vi "Test Executive.vi"(11 "Module Config":T30={"Name"="Test Executive", "Parent Q"=refnum, "Is Child?"=FALSE, "Index"=0, "Dirs"={"Root"=path "C:/MTE", "Config"=path "C:/MTE/Config", "Logs"=path "C:/MTE/Logs", "Reports"=path "C:/ATE/Reports", "App Data"=path "C:/ProgramData/Test Executive"}, "Simulate"=FALSE, "SimCtrl"=refnum}) -> ()   [LabVIEW 2018]
uses:
  <vilib>/KATE/Module/Module Config.ctl
  <vilib>/KATE/Queues/Q.Element.ctl
  <vilib>/KATE/Module/Module.Working Dirs.ctl
  Controls and Type Defs/TestExec.Station ID.ctl
  <vilib>/KATE/SeqMgr/SeqMgr.Result State Enum.ctl
  SubVIs/Metrics/TestExec.Test Result Metric Status.ctl
  Common/Utils/Results/Result.Results Table Record.ctl
  Common/Utils/Errors/Error.Error List Item.ctl
  Common/Utils/Errors/Error.Warning List Item.ctl
  Common/Utils/Results/Result XML/TestResult.SW Item.ctl
  SubVIs/TestExec.Test Result Metric History.ctl
  SubVIs/Metrics/TestExec.Test Result Metric History Item.ctl
  Controls and Type Defs/TestExec.Test Data Directories.ctl
  Common/Utils/TestExec/TestExec.WorkingDir.ctl
  Controls and Type Defs/TestExec.Options Ctrls.ctl
  <vilib>/KATE/Event Log/Event Notification/Event Log.Log Level.ctl
  Common/Utils/Results/Limits/Result.Test Limit Item.ctl
  Common/Utils/Results/Result.Limit Type.ctl
  SubVIs/Options/TestExec.Result Option Selector.ctl
  Controls and Type Defs/TestExec.Barcode PN SN Format Type.ctl
  Common/Utils/Reports/Report.Result FileDataObject.ctl
  <vilib>/KATE/Files/Sync/File.Sync Item Record.ctl
  Common/Utils/Reports/Report.Report File Config Item.ctl
  Common/Utils/Reports/Report.Report File Type.ctl
  <vilib>/KATE/Module/Module.SW Version Info.ctl
  <vilib>/KATE/Module/Window/Window.Task, Action.ctl
  Common/Utils/TestExec/TestExec.Health State Command.ctl
  SubVIs/Mode Manager/Mode Manager.lvclass
  Controls and Type Defs/TestExec.Sequence Info.ctl
  <vilib>/KATE/SeqMgr/SeqMgr.Result Info.ctl
  Controls and Type Defs/TestExec.Health Management Params.ctl
  <vilib>/KATE/SeqMgr/SeqMgr.lvclass
  <vilib>/KATE/Files/Sync/File.Sync.lvclass
  <vilib>/KATE/TCP-IP/Mgr/TCP-IP Mgr.Config.ctl
  Common/Utils/Counters/Step Counter.State Info.ctl
  Common/Utils/Results/Result.Measurement Item.ctl
  Common/Utils/Results/Result.Measurement and Attribute Item Status.ctl
  Common/Utils/Results/Result XML/TestResult.Header Info.ctl
  Common/Utils/Results/Result XML/TestResult.Facility.ctl
  Common/Utils/Results/Result XML/TestResult.Station Info.ctl
  Common/Utils/Results/Result XML/TestResult.HW Item.ctl
  Common/Utils/Results/Result XML/TestResult.Test Run Info.ctl
  Common/Utils/Results/Result XML/TestResult.Test Info.ctl
  Common/Utils/Results/Result XML/TestResult.UUT Result.ctl
  Common/Utils/Results/Result XML/TestResult.Symptom.ctl
  Common/Utils/Results/Result XML/TestResult.Symptom.State.ctl
  Common/Utils/Results/Result XML/TestResult.UUTInfo.ctl
  Common/Utils/Subscription/Subscription.Request Item.ctl
  Common/Utils/Errors/Error.Error Code List.ctl
  Common/Utils/Counters/SubVIs/Step Counter.Action.ctl
  Common/Utils/Results/Result.Attribute.ctl
  Common/Utils/Results/Result.Attribute_EV1.ctl
  Common/Utils/Results/Result XML/TestResult.FullResultData.ctl
  Common/Utils/Results/Result.Report Format Selector.ctl
  Common/Utils/Results/Result.Numeric.ctl
  Common/Utils/Results/Result.Numeric_EV1.ctl
  Common/Utils/TestExec/TestExec.Operating State.ctl
  <vilib>/KATE/Queues/Q.Msg Return Data Container.ctl
  Common/Utils/TestExec/TestExec.Test Start Message to Sta.ctl
  SubVIs/Metrics/TestExec.Test Metric Action Selector.ctl
  <vilib>/KATE/SeqMgr/SeqMgr.Result Control Ref.ctl
  <vilib>/KATE/SeqMgr/SeqMgr.Progress Controls.ctl
  Common/Utils/TestExec/TestExec.Test Launch Params.ctl
  <vilib>/KATE/Event Log/Event Notification/Event Log.Notification Type.ctl
  <vilib>/Utility/config.llb/Read Key (String).vi
  <vilib>/KATE/Config/Stored Controls/Class.SaveCtrls.lvclass
  <vilib>/KATE/Queues/Queue Utils.lvlib
  <vilib>/KATE/Module/Module Utils.lvlib
  <vilib>/KATE/Event Log/Event Log.lvlib
  <vilib>/KATE/Scheduler/Scheduler.lvlib
  <vilib>/KATE/Files/File Utils.lvlib
  <vilib>/KATE/Menu/Menu Utils.lvlib
  <vilib>/KATE/SeqMgr/SeqMgr.lvlib
  <vilib>/KATE/Config/Config Utils.lvlib
  <vilib>/KATE/Controls/Controls.lvlib
  <vilib>/KATE/Graphics/Graphic Utils.lvlib
  <vilib>/KATE/TCP-IP/TCP-IP.lvlib
  <vilib>/KATE/Event Log/Event Notification/Event Notification.lvclass
  <vilib>/KATE/Time/Time Utils.lvlib
  <vilib>/Utility/config.llb/NI_LVConfig.lvlib
  <vilib>/KATE/Config/App Data/Class.AppData.lvclass
  <vilib>/KATE/Files/Rotate/File.Rotate.lvclass
panel:
  in  "Main Tab":enum32{"Operate", "Maint"}(tab)
  in  "PersistCmt":bool caption="Persist"
  in  "Comment At End":bool caption="Prompt"
  out "Route Check":bool caption="SN Route Check"
  out "Duration(HH:MM:SS)":string
  out "Position":string
  out "Remote":bool
  out "Wiggler":bool
  out "StaCnct":bool caption="Connected"
  out "PLC":bool
  out "Status":string
  out "Result Status":T2 {"Code" format="%08d"}
  in  "Start with SN Entry":bool=TRUE caption="Start Test with SN Entry"
  in  "Go to Test Metric Details":bool
  in  "Kill Auto Launch":bool
  out "Repeat Notificaiton":string
  in  "Comment":string
  in  "SN":string
  in  "Test Result Metrics":T3
  in  "Operator":string
  in  "Mode":u16(ring) items=["Production", "Technician", "Gage R&R", "Engineering"]
  out "Station":T4
  out "End Time":timestamp format="%<%X\n%x>T"
  out "Start Time":timestamp format="%<%X\n%x>T"
  out "Simulate Indication":string="Simulating Instruments"
  in  "Funct Tab":T5(tab)
  out "Seq Rslt":string caption="Seq"
  out "SN Rslt":string caption="SN"
  in  "Test Status Tab":T6(tab)
  out "Abort Cnt":i32
  out "Test State":enum32{"Idle", "Running", "Completed"}(tab)
  out "Progress 2":dbl(slide) caption="Progress" scale=0.0..1.0
  out "Test Running 2":bool
  out "Result Status 2":T2 {"Code" format="%08d"}
  out "Yield%":dbl
  out "Error Cnt":i32
  out "Fail Cnt":i32
  out "Pass Cnt":i32
  in  "Filter":string
  in  "Show Only Failures":bool
  out "Results Table":T7[](array[typedef]) caption="Results"
  in  "Auto Scroll":bool=TRUE
  in  "Open Image File":bool
  in  "OperNo":bool
  out "OperPrompt":string caption="Oper Instructions"
  in  "OperOK":bool
  out "OperPict":picture
  in  "Zoom Img":dbl(slide)=1.0 caption="Zoom" min=0.1 max=10.0 step=0.01 scale=0.0..2.0
  in  "Zoom Right":dbl(slide)=1.0 min=0.1 max=10.0 step=0.01 scale=0.0..2.0
  in  "Zoom Left":dbl(slide)=1.0 min=0.1 max=10.0 step=0.01 scale=0.0..2.0
  out "Rigth Image":picture
  out "Left Image":picture
  in  "OperOK 2":bool
  in  "OperNo 2":bool
  in  "Prompt NO":bool
  in  "Prompt YES":bool
  in  "Prompt2_OK":bool
  in  "OperInput Data":string caption="Input Data"
  out "OperPrompt2":string caption="Instructions"
  in  "Test Reset":bool
  in  "ReportEn":T8=1 caption="Reports" items=["Enabled", "Disabled"]
  in  "Test Status Tab Sel":u16(ring) caption="View" items=["Summary", "Results", "Image1", "Image2", "Prompt"]
  out "Equipment List":string[][](table)
  in  "Health Tab":T9(tab)
  in  "Clear Errors and Warnings":bool
  in  "Clear Errors":bool
  in  "Clear Warnings":bool
  out "Warning List":T10[](array[typedef])
  out "Error List":T11[](array[typedef])
  in  "Open Event Log":bool
  in  "Open SW Version File":bool
  out "LastVerCkTime":timestamp caption="Last Version Check"
  out "SW Check Config":T12
  out "RelSWVers":string[][](array[string]) caption="Released SW Versions"
  out "Station SW Versions":T13(array[cluster])
  in  "Enable File Sync":bool=TRUE
  out "FileSyncActive":bool
  in  "Sync Now":bool
  out "Sync Items":T14[](array[typedef])
  in  "Test Metrics Tab":enum32{"Test History", "Test Reports", "Pareto"}(tab)
  in  "Test Cycle Cnt Reset":bool
  out "Total Test Cycles":i32
  in  "Test Metrics Reset":bool
  out "Test History":T15 {"Dur(s)" format="%#.1f"}
  in  "Open RprFldr":cluster{"Open":bool}[](array[cluster])
  in  "Configure Reports":bool
  out "Report Config":T17[](array[typedef]) caption="Name/\nType                                                            Sequence                                                                                             Output Folder"
  out "Pareto":i32[][](array[numeric]) caption="Code                        Count"
  in  "Config Tab":T19(tab)
  out "Force Sync Now":bool
  in  "SyncType":bool caption="Sync Type: Difference(F) or All(T)"
  in  "Set TE Sta Cfg":bool
  out "PLC Running":bool
  in  "Sim Wiggler Start":bool
  in  "TE Opts":T20={"DispDetails"=FALSE, "NotResetSN"=FALSE, "NotValOper"=FALSE, "NotValSN"=FALSE, "DisResults"=FALSE, "StaModule"=FALSE, "EditEQ"=FALSE, "ClrWarn"=FALSE, "ClrErr"=FALSE, "ViewCfg"=FALSE, "SetOpts"=FALSE, "ContOnErr"=FALSE, "ContOnFail"=TRUE, "DisMetrics"=FALSE, "SelSeq"=FALSE, "GenRpt"=FALSE, "DisStartWithSN"=FALSE, "Auto Repeat Seq En"=FALSE, "DataDirEn"=FALSE, "SNRouteCk"=FALSE} caption="TE Options"
  in  "Default Timeout (s)":dbl=1.0
  in  "Show Station Module":bool
  in  "Log Level":T21
  in  "PLC Enable":bool=TRUE
  out "Duration(s)":dbl format="%.2f"
  out "Step":string[](array[string])
  in  "Inc Step":bool
  in  "Pause":bool
  in  "Step Run":bool
  out "Script":string[][](array[string])
  out "StepCnt":i32
  in  "Run Utility":bool
  in  "Utility INI Config File":u16(ring)
  in  "Args":string[](array[string])
  in  "Exe Path":path
  in  "Run Exe":bool
  out "Seq Setup":cluster{"Name":string, "Value":string}[](array[cluster]) caption="Setup:   Name                                Value"
  out "SeqName":string caption="Name"
  out "SeqPN":string caption="PN"
  out "SeqVer":string caption="Version"
  out "Data Dir Config":T22
  out "PN":string
  out "UUT Properties":string[][](array[string])
  out "Variables":string[][](array[string])
  in  "Barcode PN SN Format":T24={"Type"=enum."SN_Only", "Len"=12, "Delimiter"="TAB"}
  out "Image Path":path
  out "Var Subscribe":bool
  in  "LoadLimFile":bool
  out "Limit File Ver":string
  out "Limits":T25[](array[typedef])
  out "Limit File Name":string
  in  "Open Root Folder":bool
  out "Cfg.Dirs":T27
  out "CfgFilePaths":T28
  out "File Data Objs":T29[](array[typedef])
  out "Title":string="Test Executive"
  out "Rev":string="v1.0.0"
  in  "Go to Health Details":bool
  out "Warnings":i32 caption="Counts"
  out "Errors":i32
  out "Health OK":bool
  out "Test Ctrl Tab":enum32{"Idle", "Running", "Completed"}(tab)
  in  "Start":bool
  out "UUT SN Status":string="Enter Operator and SN then click Start."
  in  "Sequence":u16(ring) items=["Test_01", "Test_02", "Test_03", "Test_04", "Test_05", "Test_06", "Test_07", "Test_08", "Test_09"]
  out "Test Running":bool
  out "Progress":dbl(slide) scale=0.0..1.0
  in  "Abort":bool
  out "Failing Status":string="Failing"
  in  "RepeatInt(s)":dbl=3.0 caption="(s)"
  in  "Repeat Seq":bool
  in  "Exit Sta module":bool
  out "StaModule":string
  in  "Leave Maint":bool
  out "Abort Flag":bool
  in  "Create RTF Report":bool
  out "OperCntDwn":dbl caption="Seconds Remaining" format="%#.0f"
  in  "TO_En":bool caption="Enabled"
  out "SW Items":T31[](array[typedef]) caption="This Station SW Items"
  # "Health\nStatus"
  # "Yield = 100% X Pass / (Pass + Fail + Error)"
  # "Ready\nfor Next Test"
  # "Step                                        Name                                                   Value                          Units    LimType       LL            UL           Result        Code                     Description"
  # "Image Prompt"
  # "Name                                                                            PN                                  Version                                   Checked    Wrong Version"
  # "Name                                                                     Version"
  # "Name/Interval(Hours)                                                                       Source/Destination                                                                                       Last Sync                                 Status"
  # "Dur(s)                    Time                               Mode                           Test                                   SN                               Result            Code                                          Description"
  # "Test Report Configuration"
  # "If a sequence name is listed, then the report will be sent to the corresponding folder.\nIf the sequenceis not in the list then the report will be sent to the first folder (the default folder)."
  # "Difference:    Only overwrite difference.\nAll:                    Always over write all."
  # "Sequence Info"
  # "Name                                                       Value"
  # "Name                                                       Value"
  # "String or Special Chars: \n  TAB CR LF EOL(CRLF)"
  # "Name                        Type               LL             UL                Units         FailCode                                     Fail Desc"
  # "Image1 Time Out"
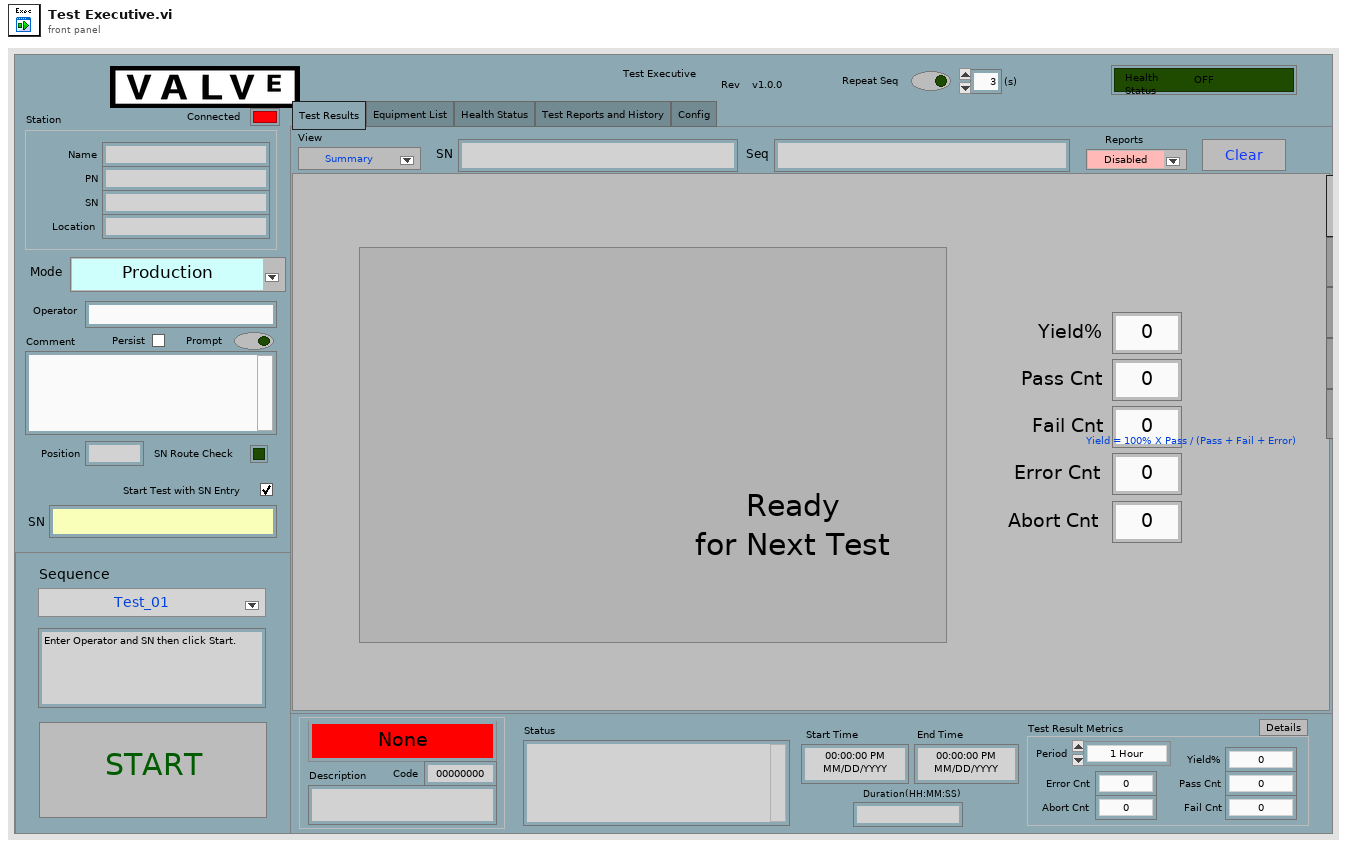
[diagram p1: front panel]
types:
  T1 = typedef "KATE_Lib.lvlib/SeqMgr.lvlib/SeqMgr.Result State Enum.ctl" = enum16{"None", "Passing", "Failing", "PASS", "FAIL", "ABORT", "ERROR"}
  T2 = cluster{"State":T1, "Code":i32, "Description":string}
  T3 = typedef "TestExec.Test Result Metric Status.ctl" = cluster{"Period":enum16{"1 Hour", "4 Hours", "1 Day", "1 Week"}, "Pass Cnt":i32, "Fail Cnt":i32, "Yield%":dbl, "Error Cnt":i32, "Abort Cnt":i32}
  T4 = typedef "TestExec.Station ID.ctl" = cluster{"Name":string, "PN":string, "SN":string, "Location":string}
  T5 = enum32{"Test Results", "Station Control", "Equipment List", "Health Status", "Test Reports and History", "Config"}
  T6 = enum32{"Summary", "Results", "Image1", "Image2", "Prompt"}
  T7 = typedef "Result.Results Table Record.ctl" = cluster{"Cnt":i32, "Step":string, "Category":string, "Name":string, "Value":string, "Units":string, "LimType":string, "LL":string, "UL":string, "Status":string, "Status Color":u32, "Code":i32, "Desc":string}
  T8 = typedef "TestExec.Result Option Selector.ctl" = u16
  T9 = enum32{"Errors/Warnings", "SW Versions", "File Sync", "File Rotation"}
  T10 = typedef "Error.Warning List Item.ctl" = cluster{"Code":i32, "Desc":string, "First":timestamp, "Last":timestamp, "Count":i32}
  T11 = typedef "Error.Error List Item.ctl" = cluster{"Code":i32, "Desc":string, "First":timestamp, "Last":timestamp, "Count":i32}
  T12 = cluster{"Check Interval":dbl, "SW Version List File":path, "Enabled":bool}
  T13 = cluster{"Name":string, "PN":string, "Version":string, bool, bool}[]
  T14 = typedef "KATE_Lib.lvlib/File Utils.lvlib/File.Sync.lvclass/File.Sync Item Record.ctl" = cluster{"Name":string, "Interval":dbl, "Source":path, "Dest":path, "LastSync":timestamp, "Status":string, "Error":bool, "Type":enum16{"Merge", "Match"}}
  T15 = typedef "TestExec.Test Result Metric History.ctl" = T16[]
  T16 = typedef "TestExec.Test Result Metric History Item.ctl" = cluster{"TimeStamp":timestamp, "Dur(s)":dbl, "Time":string, "Mode ":string, "Test ":string, "SN":string, "State":T1, "Code":i32, "Description":string}
  T17 = typedef "Report.Report File Config Item.ctl" = cluster{"Name":string, "Type":T18, "Seq_Dir":cluster{"Sequence":string, "Folder":path}[]}
  T18 = typedef "Report.Report File Type.ctl" = enum16{"CSV_WithConfigAndData", "CSV", "CSV_SummaryResult", "JSON", "JSON_WithFiles", "XLINK", "XLINK_ResultOnly", "SFC1", ""}
  T19 = enum32{"Options", "Script Debug", "Run Util", "Run Exe", "Client Info", "Local Data", "Limits", "Dirs", "File Objs"}
  T20 = typedef "TestExec.Options Ctrls.ctl" = cluster{"DispDetails":bool, "NotResetSN":bool, "NotValOper":bool, "NotValSN":bool, "DisResults":bool, "StaModule":bool, "EditEQ":bool, "ClrWarn":bool, "ClrErr":bool, "ViewCfg":bool, "SetOpts":bool, "ContOnErr":bool, "ContOnFail":bool, "DisMetrics":bool, "SelSeq":bool, "GenRpt":bool, "DisStartWithSN":bool, "Auto Repeat Seq En":bool, "DataDirEn":bool, "SNRouteCk":bool}
  T21 = typedef "KATE_Lib.lvlib/Event Log.lvlib/Event Log.Log Level.ctl" = enum16{"Normal", "Verbose", "Debug0", "Debug1", "Debug2"}
  T22 = typedef "TestExec.Test Data Directories.ctl" = cluster{"Station Data":T23[], "SeqRsltDirs":T23[]}
  T23 = typedef "TestExec.WorkingDir.ctl" = cluster{"Name":string, "Path":path}
  T24 = typedef "TestExec.Barcode PN SN Format Type.ctl" = cluster{"Type":enum16{"SN_Only", "SN_PN_LenDelim", "PN_SN_LenDelim", "SN_PN_StrDelim", "PN_SN_StrDelim"}, "Len":i32, "Delimiter":string}
  T25 = typedef "Result.Test Limit Item.ctl" = cluster{"Name":string, "LimType":T26, "LL":string, "UL":string, "Units":string, "FailCode":i32, "FailDesc":string}
  T26 = typedef "Result.Limit Type.ctl" = enum16{"None", "EQ", "NE", "GT", "LT", "GE", "LE", "GTLT", "GELE", "GELT", "GTLE", "LTGT", "LEGE", "LEGT", "LTGE", "Contains", "NotContains"}
  T27 = typedef "KATE_Lib.lvlib/Module Utils.lvlib/Module.Working Dirs.ctl" = cluster{"Root":path, "Config":path, "Logs":path, "Reports":path, "App Data":path}
  T28 = cluster{"ModeCfg":path, "DataTemp":path, "SW Limits":path, "SW Sequences":path, "Rel_SW":path, "Current Seq Dir":path, "RouteCfg":path, "WorkingCfg":path, "Devcon":path, "ScriptLibDirs":path[], "Archive":path, "LocalData":path}
  T29 = typedef "Report.Result FileDataObject.ctl" = cluster{"Cnt":i32, "Step":string, "Category":string, "Name":string, "Type":string, "File Name":string, "Time":string, "Path":path}
  T30 = typedef "KATE_Lib.lvlib/Module Utils.lvlib/Module Config.ctl" = cluster{"Name":string, "Parent Q":refnum<queue>, "Is Child?":bool, "Index":i32, "Dirs":T27, "Simulate":bool, "SimCtrl":refnum<vi>}
  T31 = typedef "TestResult.SW Item.ctl" = cluster{"Name":string, "PN":string, "Version":string, "Note":string}
  T32 = typedef "KATE_Lib.lvlib/Module Utils.lvlib/Module.SW Version Info.ctl" = cluster{"AppName":string, "Company":string, "Version":string, "Description":string, "PN":string}
  T33 = typedef "KATE_Lib.lvlib/Module Utils.lvlib/Module Sys Info.ctl" = cluster{"Main Q":refnum<queue>, "Exe":bool, "SW Rev":T32, "Self Ref":refnum<vi>, "Main Tab":refnum<vi>, "Pane":refnum<vi>, "Stop":cluster{"Ref":refnum<event-registration>, "Event":refnum<user-event>}, "Cfg":T30, "Services":cluster{"Name":string, "vi ref":refnum<vi>}[], "Menu Ref":refnum<k9>, "CtrlStates":refnum<class "Class.SaveCtrls.lvclass">, "Docs":cluster{"Tags":string[], "Paths":path[]}, "Log":refnum<class "Event Notification.lvclass">, "Test Controls":refnum<vi>[], "Child Modules":cluster{"Name":string, "vi ref":refnum<vi>}[], "SW Items":string[][], "AppData":refnum<class "Class.AppData.lvclass">, "Subscriptions":refnum<class "Subscription.lvclass">}
  T34 = typedef "KATE_Lib.lvlib/TCP-IP.lvlib/TCP-IP Mgr.Config.ctl" = cluster{"IP":string, "Port":u16, "Listener":bool, "Enable":bool}
  T35 = cluster{"Oper":cluster{"OK":bool, "Desc":string}, "SN":cluster{"OK":bool, "Desc":string}, "NoSN":bool, "DefaultSN":string, "SNErr":bool, "SeqEn":enum8{"Enabled", "Disabled", "Disabled and Grayed Out"}}
  T36 = enum8{"Enabled", "Disabled", "Disabled and Grayed Out"}
  T37 = typedef "TestExec.Health State Command.ctl" = enum16{"Update", "Clear All", "Clear Warnings", "Clear Errors", "Set Warning", "Set Error"}
  T38 = typedef "Result.Measurement Item.ctl" = cluster{"Cnt":i32, "Step":string, "Category":string, "Name":string, "Value":string, "Units":string, "LimType":string, "LL":string, "UL":string, "Status":T39, "Code":i32, "Desc":string, "Time":timestamp}
  T39 = typedef "Result.Measurement and Attribute Item Status.ctl" = i32
  T40 = typedef "Step Counter.Action.ctl" = enum16{"Init", "Section Start", "Data +", "Sub Section Start", "Sub Section End", "Get Step"}
  T41 = typedef "TestResult.HW Item.ctl" = cluster{"Name":string, "MFG":string, "PN":string, "SN":string, "SW/FW":string, "Note":string, "Cal_ID":string, "Cal_Type":string, "Cal_Due_Date":timestamp, "Cal_Status":string}
  T42 = cluster{"Config Folder":path, "Seq Folder":path, "Rel SW File":path, "SW Check Int(s)":dbl, "Vers":variant, "SW Check En":bool}
  T43 = typedef "Result.Attribute.ctl" = cluster{"Cnt":i32, "Step":string, "Category":string, "Name":string, "Value":string, "Status":T39, "Code":i32, "Desc":string, "Time":timestamp}
  T44 = typedef "Result.Attribute_EV1.ctl" = cluster{"Cnt":i32, "Step":string, "Category":string, "Name":string, "Value":string, "Status":T39, "Code":i32, "Desc":string}
  T45 = typedef "Result.Report Format Selector.ctl" = enum16{"XML", "CSV", "Xlink XML", "XML with Files", "JSON", "JSON with Files", "RTF", "SFC1"}
  T46 = typedef "TestResult.FullResultData.ctl" = cluster{"#attributes":cluster{"Version":string}, "Station":T47, "Test Run":T48, "Test Sequence":T49, "UUTs":cluster{"UUT":T50[]}}
  T47 = typedef "TestResult.Station Info.ctl" = cluster{"Name":string, "PN":string, "SN":string, "Rev":string, "PC Name":string, "Location":string, "HW_Config":cluster{"HW_Item":T41[]}, "SW_Config":cluster{"SW_Item":T31[]}}
  T48 = typedef "TestResult.Test Run Info.ctl" = cluster{"Operator":string, "Start Time":timestamp, "Duration(s)":dbl, "Mode":string, "Comment":string, "ProcessStep":string}
  T49 = typedef "TestResult.Test Info.ctl" = cluster{"Name":string, "Config":cluster{"Config_Item":cluster{"Name":string, "Value":string}[]}}
  T50 = typedef "TestResult.UUT Result.ctl" = cluster{"Position":string, "Result":T51, "Measurements":cluster{"Measurement":T38[]}, "UUTInfo":T53}
  T51 = typedef "TestResult.Symptom.ctl" = cluster{"Result":T52, "Code":i32, "Description":string}
  T52 = typedef "TestResult.Symptom.State.ctl" = enum16{"Pass", "Fail", "Error", "Aborted", "Completed", "Logged"}
  T53 = typedef "TestResult.UUTInfo.ctl" = cluster{"Product":string, "Desc":string, "PN":string, "SN":string, "Lot":string, "DateCode":string, "AltID":string, "Revision":string, "Properties":cluster{"Property":cluster{"Name":string, "Value":string}[]}}
  T54 = typedef "TestExec.Operating State.ctl" = cluster{"Test State":enum32{"Idle", "Running", "Completed"}, "Result":T1, "Sequence":string, "Sequences":string[], "SN":string, "Position":string}
  T55 = typedef "KATE_Lib.lvlib/Queue Utils.lvlib/Q.Msg Return Data Container.ctl" = cluster{"SeqNum":i32, "Data":variant, "Error":errorcluster}
  T56 = typedef "TestExec.Test Start Message to Sta.ctl" = cluster{"Test Name":string, "Start Time":timestamp, "UUT SN":string}
  T57 = typedef "KATE_Lib.lvlib/Module Utils.lvlib/Window.Task, Action.ctl" = enum16{"Resize()", "Show Panel(Bool)", "Show Scroll Bars(Bool)", "Dock to SubPanel(SubPanel Ref)", "Undock from SubPanel()", "Return to SubPanel()", "Go To Maint Tab()", "Show Maint Tab(Bool)", "Open Block Diagram()"}
  T58 = typedef "Subscription.Request Item.ctl" = cluster{"Name":string, "Msg":T59}
  T59 = typedef "KATE_Lib.lvlib/Queue Utils.lvlib/Q.Element.ctl" = cluster{"Cmd":string, "Sub":string, "Data1":variant, "Data2":variant}
  T60 = typedef "TestExec.Test Metric Action Selector.ctl" = enum16{"Append", "Get Metrics", "Reset", "Load", "Save"}
  T61 = typedef "TestExec.Test Launch Params.ctl" = cluster{"Sequence":string, "SN":string, "Pos":string}
  T62 = cluster{"Config_Item":cluster{"Name":string, "Value":string}[]}
  T63 = typedef "KATE_Lib.lvlib/SeqMgr.lvlib/SeqMgr.Result Info.ctl" = cluster{"State":T1, "Code":i32, "Description":string}
  T64 = typedef "KATE_Lib.lvlib/Event Log.lvlib/Event Log.Notification Type.ctl" = enum16{"Normal", "Warning", "Error", "Success"}
  T65 = typedef "TestExec.Health Management Params.ctl" = cluster{"Warnings":i32, "Errors":i32, "LastVerCk":dbl, "VerCkInterval":dbl, "SW Check En":bool, "Init":bool, "LastVerListCk":dbl}
  T66 = typedef "TestExec.Sequence Info.ctl" = cluster{"Name":string, "Path":path}
  T67 = cluster{"ModeCfg":path, "DataTemp":path, "SW Limits":path, "SW Sequences":path, "Rel_SW":path, "CurSeqDir":path, "RouteCfg":path, "WorkingCfg":path, "Devcon":path, "ScriptLibDirs":path[], "Archive":path, "LocalData":path}
  T68 = cluster{"Child Modules":cluster{"VI Ref":refnum<vi>, "Name":string}[]}
  T69 = cluster{"Limits":variant, "Limit File":string, "Limit Ver":string, "RsltCodes":variant, "Rslt Code File":string, "Rslt Code Ver":string, "Default Seq":i32, "FaultPrefix":i32, "UUTRoutes":string[], "DisableRouteCk":bool, "StaVer":i32, "SN Valid":bool, "ReqVars":bool, "Product":string, "ProcessStep":string, "FileSyncMaster":path, "CmtPrmpt":bool}
  T70 = typedef "TestResult.Header Info.ctl" = cluster{"#attributes":cluster{"Version":string}, "Facility":T71, "Station":T47, "Test Run":T48, "Test Sequence":T49}
  T71 = typedef "TestResult.Facility.ctl" = cluster{"Name":string, "Location":string}
  T72 = typedef "Step Counter.State Info.ctl" = cluster{"Level":i32, "Cnts":i32[], "Step":string, "Cntr":i32}
  T73 = cluster{"Lnch":bool, "SeqTimer":dbl, "TimeOut(s)":dbl, "ModeMgr":refnum<class "Mode Manager.lvclass">, "CfgFilePaths":cluster{"ModeCfg":path, "DataTemp":path, "SW Limits":path, "SW Sequences":path, "Rel_SW":path, "CurSeqDir":path, "RouteCfg":path, "WorkingCfg":path, "Devcon":path, "ScriptLibDirs":path[], "Archive":path, "LocalData":path}, "Data Dirs":T22, "StaApp":string, "App":cluster{"Child Modules":cluster{"VI Ref":refnum<vi>, "Name":string}[]}, "Sequences":T66[], "PreTestCk":cluster{"Oper":cluster{"OK":bool, "Desc":string}, "SN":cluster{"OK":bool, "Desc":string}, "NoSN":bool, "DefaultSN":string, "SNErr":bool, "SeqEn":enum8{"Enabled", "Disabled", "Disabled and Grayed Out"}}, "Seq":string[][], "SeqMgr":refnum<class "SeqMgr.lvclass">, "Health":T65, "ResultState":T63, "SW_Vers":variant, "Repeat(s)":dbl, "DisableResults":bool, "SectCtr":T72, "Data":cluster{"FileObjs":T29[], "Meas":T38[]}, "ResultError":errorcluster, "RptHdr":T70, "RptUUT":T50, "Lists":cluster{"Limits":variant, "Limit File":string, "Limit Ver":string, "RsltCodes":variant, "Rslt Code File":string, "Rslt Code Ver":string, "Default Seq":i32, "FaultPrefix":i32, "UUTRoutes":string[], "DisableRouteCk":bool, "StaVer":i32, "SN Valid":bool, "ReqVars":bool, "Product":string, "ProcessStep":string, "FileSyncMaster":path, "CmtPrmpt":bool}, "TestCanceled":bool, "Opts":T20, "UUT Dir":path, "Funct":cluster{"Seq":i32, "Name":string}, "StaNotify":bool, "Subscr":T58[], "Sync":refnum<class "File.Sync.lvclass">, "RptCfg":T17[]}
  T74 = typedef "Error.Error Code List.ctl" = i32
  T75 = cluster{"Name":string, "PN":string, "Version":string, bool, bool}
  T76 = typedef "ModeMgr.Mode Settings.ctl" = cluster{"Option":string, "Level":i32}
  T77 = typedef "Result.Numeric.ctl" = cluster{"Cnt":i32, "Step":string, "Category":string, "Name":string, "Value":dbl, "Units":string, "LimType":T26, "LL":dbl, "UL":dbl, "Status":T39, "Code":i32, "Desc":string, "Time":timestamp}
  T78 = typedef "Result.Numeric_EV1.ctl" = cluster{"Cnt":i32, "Step":string, "Category":string, "Name":string, "Value":dbl, "Units":string, "LimType":T26, "LL":dbl, "UL":dbl, "Status":T39, "Code":i32, "Desc":string}
  T79 = cluster{"Name":string, "Image":path, "Timeout":bool, "OK":bool}
  T80 = cluster{"Left":path, "Right":path, "Result":T43, "OK":bool, "Zoom":dbl}
  T81 = cluster{"Vars":string[][], "Items":string[][], "Path":path, "Exists":bool}
  T82 = typedef "NI_LVConfig.lvlib/Config Data RefNum.ctl" = refnum<k1>
  T83 = typedef "TestExec.Local Result Data.ctl" = cluster{"Attr":T43[], "Num":T77[], "UUT Props":string[][], "Vars":string[][], "SW Items":T31[], "Error":errorcluster, "Step":i32, "FileObjs":T29[], "MeasData":T38[]}
  T84 = typedef "KATE_Lib.lvlib/SeqMgr.lvlib/SeqMgr.Progress Controls.ctl" = cluster{"Running":refnum<vi>, "StartTime":refnum<vi>, "EndTime":refnum<vi>, "ProgressBar":refnum<vi>, "Duration(s)":refnum<vi>, "Test Ctrl Tab":refnum<vi>, "Failing Status":refnum<vi>}
  T85 = typedef "KATE_Lib.lvlib/SeqMgr.lvlib/SeqMgr.Result Control Ref.ctl" = cluster{"State":refnum<vi>, "Code":refnum<vi>, "Desc":refnum<vi>, "StateColors":u32[]}
  T86 = typedef "PLC.Type.ctl" = enum16{"None", "Dial 750", "Dial 800"}
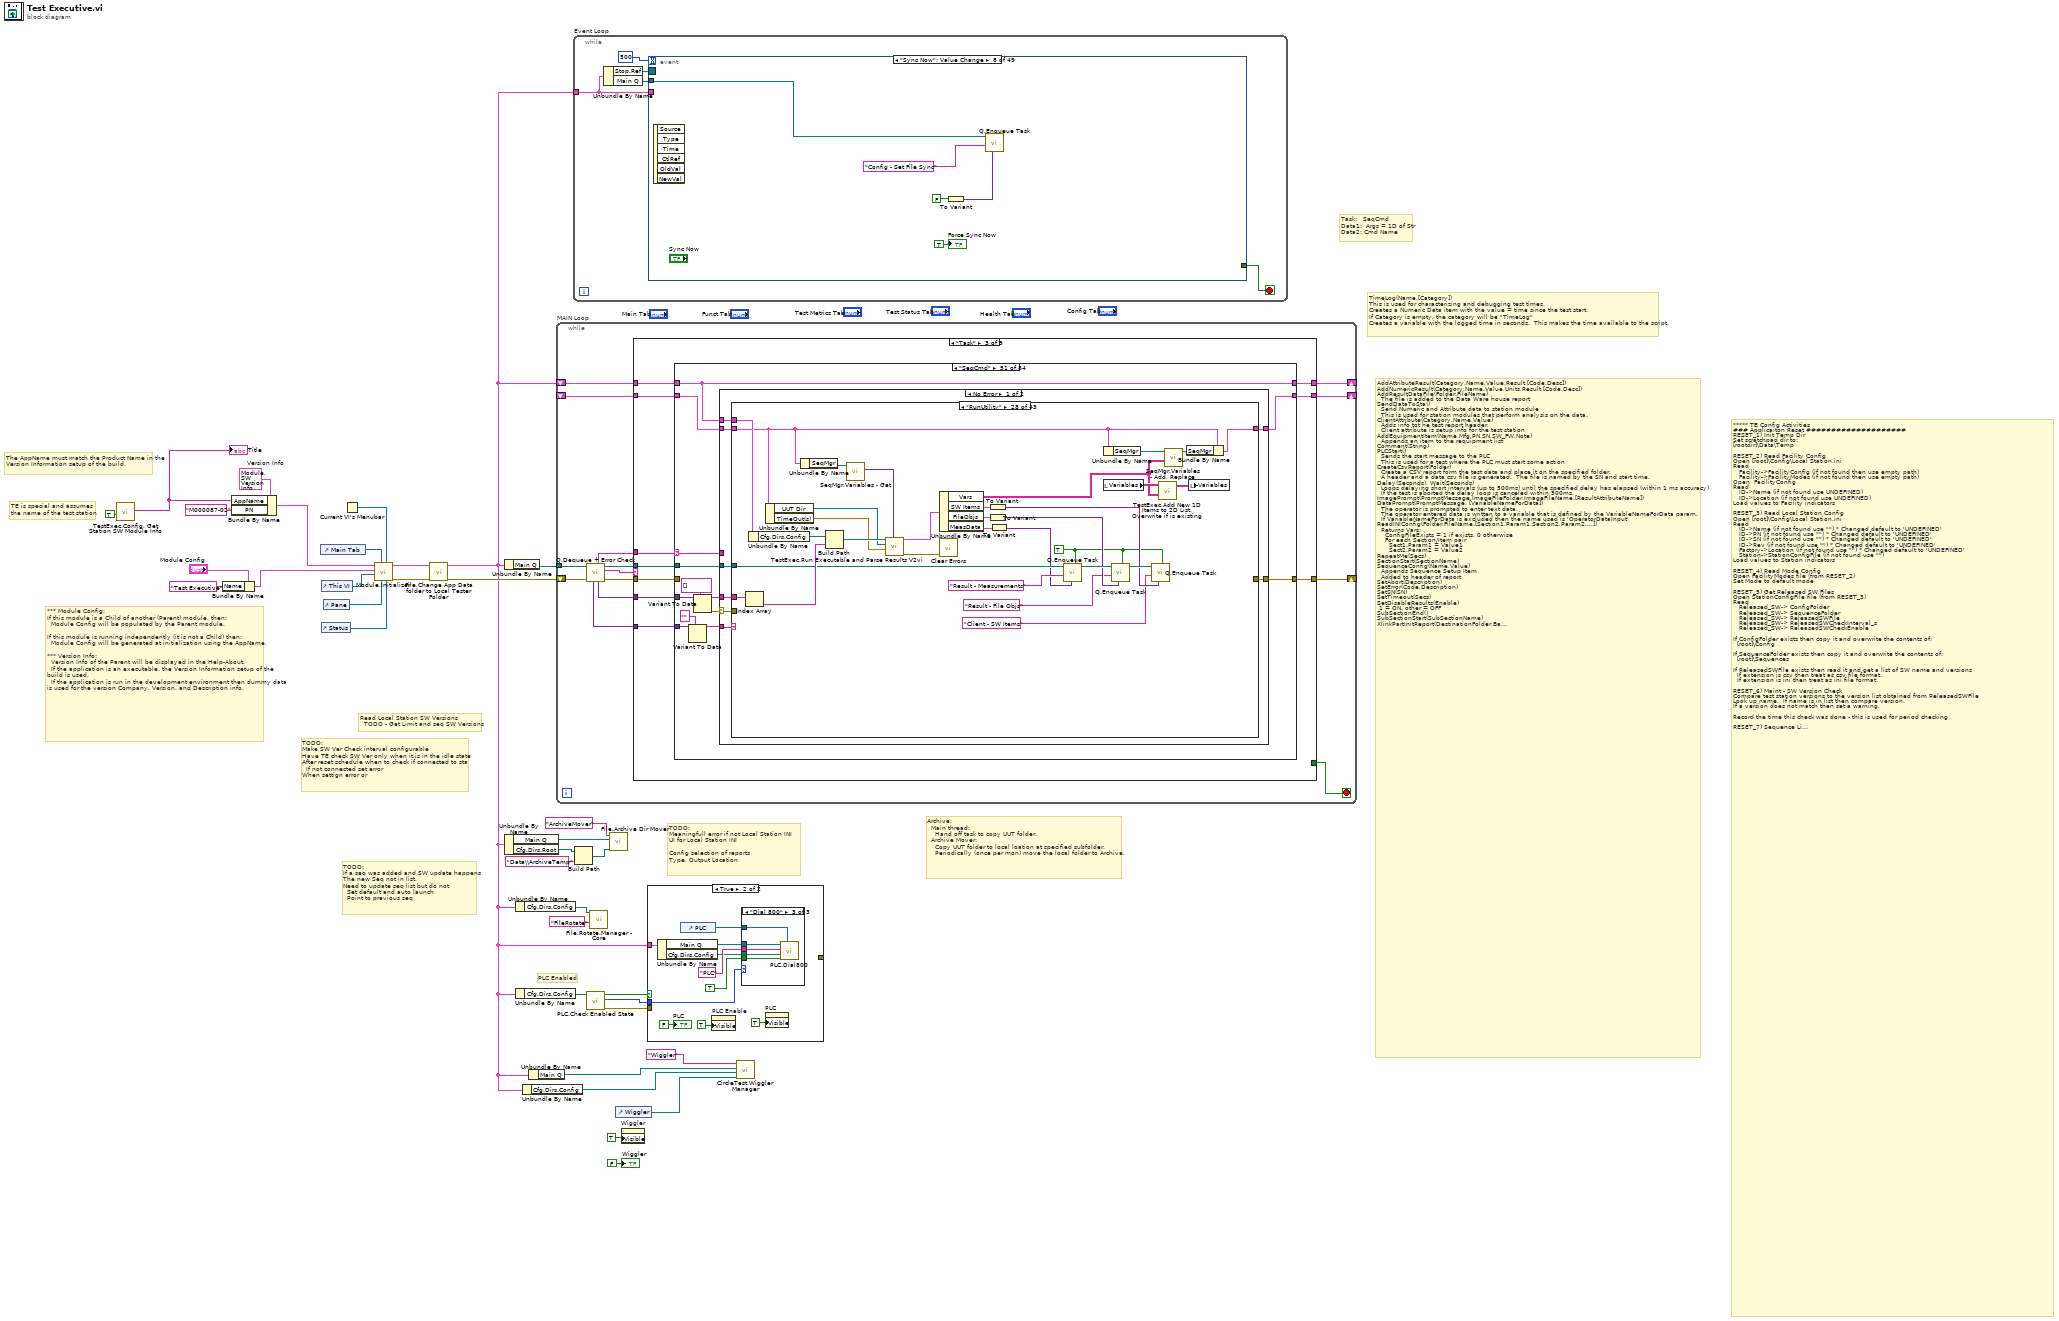
[diagram p0: block diagram]
diagram:
  w26 = T32 {"AppName"="ModuleX", "Company"="CompanyX", "Version"="1.0", "Description"="This app is being developed.", "PN"=""}  # Version Info
  # "Archive:\n  Main thread:  \n    Hand off task to copy UUT folder.\n  Archive Mover:\n    Copy UUT folder to local loation at specified subfolder.\n    Periodically (once per mon) move the local folder to Archive."
  # "TODO:\nMeaningfull error if not Local Station INI\nUI for Local Station INI\n\nConfig selection of reports\nType, Output Location"
  # "Task:   SeqCmd\nData1:  Args = 1D of Str\nData2: Cmd Name"
  # "TimeLog(Name,[Category])\nThis is used for characterizing and debugging test times. \nCreates a Numeric Data item with the value = time since the test start.\nIf Category is empty, the category will be \"TimeLog\"\nCreates a variable with the logged time in seconds.  This makes the time available to the script."
  # "TODO:\nIf a seq was added and SW update happens\nThe new Seq not in list.\nNeed to update seq list but do not \n  Set default and auto launch\n  Point to previous seq"
  # "***** TE Config Activities\n### Applicaiton Reset ####################\nRESET_1) Init Temp Dir\nSet scratchpad dir to:\n[rootdir]\\Data\\Temp\n\nRESET_2) Read Facility Config\nOpen [root]\\Config\\Local Station.ini\nRead\n   Facility->FacilityConfig (if not found then use empty path)\n   Facility->FacilityModes (if not found then use empty path)\nOpen  FacilityConfig\nRead \n   ID->Name (if not found use UNDEFINED)\n   ID->Location (if not found use UNDEFINED)\nLoad values to Facility indicators\n\nRESET_3) Read Local Station Config\nOpen [root]\\Config\\Local Station.ini\nRead\n   ID->Name (if not found use \"\") * Changed default to 'UNDEFINED'\n   ID->PN (if not found use \"\") * Changed default to 'UNDEFINED'\n   ID->SN (if not found use \"\") * Changed default to 'UNDEFINED'\n   ID->Rev (if not found use \"\") * Changed default to 'UNDEFINED'\n   Factory->Location (if not found use \"\") * Changed default to 'UNDEFINED'\n   Station->StationConfigFile (if not found use \"\")\nLoad values to Station indicators\n\nRESET_4) Read Mode Config\nOpen FacilityModes file (from RESET_2)\nSet Mode to default mode\n\nRESET_5) Get Released SW Files\nOpen StationConfigFile file (from RESET_3)\nRead\n   Released_SW-> ConfigFolder\n   Released_SW-> SequenceFolder\n   Released_SW-> ReleasedSWFile\n   Released_SW-> ReleasedSWCheckInterval_s\n   Released_SW-> ReleasedSWCheckEnable\n\nIf ConfigFolder exists then copy it and overwrite the contents of:\n  [root]\\Config\n\nIf SequenceFolder exists then copy it and overwrite the contents of:\n  [root]\\Sequences\n\nIf ReleasedSWFile exists then read it and get a list of SW name and versions\n  If extension is csv then treat as csv file format.\n  If extension is ini then treat as ini file format.\n\nRESET_6) Maint - SW Version Check\nCompare test station versions to the version list obtained from ReleasedSWFile\nLook up name.  If name is in list then compare version.\nIf a version does not match then set a warning.\n\nRecord the time this check was done - this is used for period checking\n\nRESET_7) Sequence List\nCreate a list of sequences form the folder names in:\n   [root]\\Sequences\n\nRESET_8) Read Result Data Dir Config\nRead StationConfigFile (from RESET_3)\nCreate a Name/Value list of the items in the section 'DataDirs'\n\nThe item named ResultsLocalDir will be used by TE for Factorylogix XML files.\nThe item named ResultsExternalDir will be used by TE for Data Warehouse XML files.\nOther items will be kept in the list.\n\nThis list of folders is forwarded to the Station Module.\nThe only module that uses this list is Circle Test.\n  It stores config and archive files in these folders.\n  It hands off data form Captue to Solve in these folders\n\n \n### Periodic Maintenance ####################\nMAINT_1) When the test station is idle and if ReleasedSWCheckEnable it calls the 'Maint - Scheduler' task\n\nMAINT_2) Maint - Scheduler\nThe last time the check was performed (initialized in step RESET_6 and reset in MAINT_2) is checked.\nIf maintenance is due it calls:\na. Get Released SW Files\nb. Maint - SW Version Check\nThe maint check timer is reset\n\n### Sequence Start ####################\n1) Load the Sequence File\n2) Read Limit File\nFirst look in the folder of the current sequence.  \nIf not found then look in the station limit config folder:\n   [root]\\Config\\Limits\\\nLook for the first file matching the pattern: Test Limits*.xml"
  # "AddAttributeResult(Category,Name,Value,Result,[Code,Desc])\nAddNumericResult(Category,Name,Value,Units,Result,[Code,Desc])\nAddResultDataFile(Folder,FileName)\n  The file is added to the Data Ware house report\nSendDataToSta()\n  Send Numeric and Attribute data to station module\n  This is used for station modules that perform analysis on the data.\nClientAttribute(Category,Name,Value)\n  Adds info tot he test report header.\n  Client attribute is setup info for the test station\nAddEquipmentItem(Name,Mfg,PN,SN,SW_FW,Note)\n  Appends an item to the requipment list\nComment(String)\nPLCStart()\n  Sends the start message to the PLC\n  This is used for a test where the PLC must start some action\nCreateCsvReport(Folder)\n  Create a CSV report form the test data and place it on the specified folder.\n  A header and a data csv file is generated.  The file is named by the SN and start time.\nDelay(Seconds), Wait(Seconds)\n  Loops delaying short intervals (up to 500ms) until the specified delay has elapsed (within 1 ms accuracy) \n  If the test is aborted the delay loop is canceled within 500ms.\nImagePrompt(PromptMessage,ImageFileFolder,ImageFileName,[ResultAttributeName])\nDataPrompt(PromptMessage, [VariableNameForData])\n  The operator is prompted to enter text data.\n  The operator entered data is written to a variable that is defined by the VariableNameForData param.\n  If VariableNameForData is excluded then the name used is 'OperatorDataInput'\nReadINIConfig(Folder,FileName,[Section1,Param1,Section2,Param2,...])\n  Returns Vars:\n    ConfigFileExists = 1 if exists, 0 otherwise\n    For each Section/Item pair \n      Sect1.Param1 = Value1\n      Sect2.Param2 = Value2\nRepeatMe(Secs)\nSectionStart(SectionName)\nSequenceConfig(Name,Value)\n  Appends Sequence Setup Item\n  Added to header of report\nSetAbort(Description)\nSetError(Code,Description)\nSetSN(SN)\nSetTimeout(Secs)\nSetDisableResults(Enable)\n 1 = ON, other = OFF\nSubSectionEnd()\nSubSectionStart(SubSectionName)\nXlinkPartInitReport(DestinationFolder,Batch,Name)\n\nMath\nAssign Var\nGetTimer(VarName [, Timer#])\n    Selects Timer#.  If this param is omitted then it used Timer0\n    Write the timer value to VarName\n    The value is:\n      Time since the timer was reset.\n      Timers are all reset at start of test.\nInitTimer([Timer#])\n    Sets Timer to now.\n    If no param then will use timer0\nSetFail(Code,Description)\nSetStopOnFail()\n 1 = ON, other = OFF\nEnd(Enable)\n Ends the sequence if the param is 1\n  Otherwise do nothing\nCancelTest()\n  Ends the test adn does not record any results\nGoTo(Label)\n  Goes to the specified label\n  A label is a line int he text that contains a string followed by a colon\nIf   Else   End If\nWhile     End While\nFor  Next"
  # "TE is special and assumes \nthe name of the test station"
  # "*** Module Config:\nIf this module is a Child of another (Parent) module, then:\n  Module Config will be populated by the Parent module.\n\nIf this module is running independently (it is not a Child) then:\n  Module Config will be generated at initialization using the AppName.\n\n*** Version Info:\n  Version Info of the Parent will be displayed in the Help-About.\n  If the application is an executable, the Version Information setup of the build is used.\n  If the application is run in the development environment then dummy data is used for the version Company, Version, and Description info."
  # "The AppName must match the Product Name in the Version Information setup of the build."
  # "Read Local Station SW Versions\n  TODO - Get Limit and seq SW Versions"
  # "TODO:\nMake SW Ver Check interval configurable\nHave TE check SW Ver only when it is in the idle state \nAfter reset schedule when to check if connected to sta\n  If not connected set error\nWhen settign error or"
  # "PLC Enabled"
  n1 = call "TestExec.Config, Get Station SW Module Info.vi"("Create File if Doesn't Exist"=TRUE) -> ("Station Name"=w21:string)  [unwired: 7 in, 3 out]
  "Title" <- w21
  n2 = Bundle By Name(cluster="Module Config", "Name"="Test Executive" ("AppName")) -> (w23:T30)
  n3 = Bundle By Name(cluster=w26, "AppName"=w21, "PN"="M000087-02") -> (w25:T32)
  n4 = control-ref of="Main Tab"() -> (w32:refnum<vi>)
  n5 = control-ref of="This VI"() -> (w31:refnum<vi>)
  n6 = control-ref of="Status"() -> (w27:refnum<vi>)
  n7 = control-ref of="Pane"() -> (w30:refnum<vi>)
  n8 = Current VI's Menubar() -> (w29:refnum<k9>)
  n9 = call <vilib>:"Module.Initializer.vi"("StatusTxtBx"=w27, "Menu Ref"=w29, "Pane"=w30, "Main Tab"=w32, "Self Ref"=w31, "Module Config"=w23, "SW Rev"=w25) -> ("error out"=w34:errorcluster, "Sys"=w5:T33)  [unwired: 3 in]
  n10 = call "File.Change App Data folder to Local Tester Folder.vi"("Sys"=w5) -> ("Sys Out"=w4:T33)  [unwired: 9 in, 1 out]
  n11 = Unbundle By Name(w4) -> ("Main Q"=w33:refnum<queue>)
  n12 = Unbundle By Name(w4) -> ("Main Q"=w8:refnum<queue>, "Cfg.Dirs.Root"=w3:path)
  n13 = Unbundle By Name(w4) -> ("Cfg.Dirs.Config"=w6:path)
  n14 = Unbundle By Name(w4) -> ("Cfg.Dirs.Config"=w28:path)
  n15 = Unbundle By Name(w4) -> ("Cfg.Dirs.Config"=w13:path)
  n16 = Unbundle By Name(w4) -> ("Main Q"=w14:refnum<queue>)
  n17 = while "MAIN Loop" {
    shift-right: [w45] -> _
    shift-left: w34 -> [w43]
    shift-right: [w46] -> _
    shift-left: _ -> [w48]
    shift-right: [w47] -> _
    shift-left: w4 -> [w37]
    tunnel: w33 -> [w42]
    stop <- w38 stop-if-true
    n18 = call <vilib>:"Q.Dequeue + Error Check.vi"("Error In"=w43, "Q In"=w42) -> ("error out"=w44:errorcluster, "Cmd"=w36:string, "Q Out"=w41:refnum<queue>, "Data1"=w40:variant, "Sub"=w35:string, "Data2"=w39:variant)  [unwired: 4 in]
    n19 = case shown="\"Task\"" w36 {
      selector: w36 -> [_ _ _ _ _ _ _ w5254 _]
      tunnel: w48 -> [_ w336 w461 w4320 w4327 w5062 w5074 w5249 w5285]
      tunnel: w37 -> [w83 w335 w462 w4321 w4329 w5063 w5076 w5256 w5283]
      tunnel: [w84 w335 w460 w4321 w4328 w5061 w5075 w5256 w5283] -> w47
      tunnel: [w74 w339 w459 w4320 w4326 w5060 w5073 w5248 w5285] -> w46
      tunnel: [w58 w330 w453 _ _ w5055 w5071 w5255 w5287] -> w45
      tunnel: w44 -> [w88 w337 w455 _ _ w5056 _ w5252 _]
      tunnel: w41 -> [w89 w338 w456 _ w4324 w5057 w5069 w5250 _]
      tunnel: w40 -> [_ _ w457 _ w4323 w5058 w5072 w5253 _]
      tunnel: w39 -> [_ _ w454 _ w4322 w5054 w5068 _ _]
      tunnel: w35 -> [_ _ w458 w4319 w4325 w5059 w5070 w5251 _]
      tunnel: [_ _ _ _ _ _ _ _ TRUE] -> w38
      frame "Init" {
        # "Use this name for communicating\nto Station app"
        n20 = call <vilib>:"Q.Enqueue Reset.vi"("Error In"=w88, "Q In"=w89) -> ("Q Out"=w78:refnum<queue>)  [unwired: 8 in, 1 out]
        n21 = stacked-sequence {
          tunnel: [_ _ w132 _ _ _ _ _ _ _ _] -> w87
          tunnel: [_ _ w136 _ _ _ _ _ _ _ _] -> w86
          tunnel: [_ _ w144 _ _ _ _ _ _ _ _] -> w85
          tunnel: w83 -> [w90 w116 _ w161 w208 _ _ w293 w301 _ w314]
          tunnel: [_ _ w143 _ _ _ _ _ _ _ _] -> w82
          tunnel: [_ _ w135 _ _ _ _ _ _ _ _] -> w81
          tunnel: [_ _ w142 _ _ _ _ _ _ _ _] -> w76
          tunnel: [_ _ _ _ w207 _ _ _ _ _ _] -> w80
          tunnel: [_ _ _ w167 _ _ _ _ _ _ _] -> w79
          tunnel: w78 -> [_ _ _ w163 _ w236 _ _ _ _ _]
          tunnel: [_ _ _ w157 _ _ _ _ _ _ _] -> w58
          tunnel: [_ _ w145 _ _ _ _ _ _ _ _] -> w77
          tunnel: [_ _ _ w146 _ _ _ _ _ _ _] -> w73
          tunnel: [_ _ w141 _ _ _ _ _ _ _ _] -> w72
          tunnel: [_ _ w140 _ _ _ _ _ _ _ _] -> w71
          tunnel: [_ _ w139 _ _ _ _ _ _ _ _] -> w70
          tunnel: [_ _ w134 _ _ _ _ _ _ _ _] -> w69
          tunnel: [_ _ w137 _ _ _ _ _ _ _ _] -> w68
          tunnel: [_ _ w138 _ _ _ _ _ _ _ _] -> w67
          tunnel: [_ _ _ _ _ w231 _ _ _ _ _] -> w66
          tunnel: [_ _ _ _ _ w239 _ _ _ _ _] -> w65
          tunnel: [_ _ _ _ _ w247 _ _ _ _ _] -> w64
          tunnel: [_ _ _ _ _ w245 _ _ _ _ _] -> w63
          tunnel: [_ _ _ _ _ w244 _ _ _ _ _] -> w62
          tunnel: [_ _ _ _ _ w246 _ _ _ _ _] -> w61
          tunnel: [_ _ _ _ _ w242 _ _ _ _ _] -> w60
          tunnel: [_ _ _ _ _ w243 _ _ _ _ _] -> w59
          tunnel: [_ _ _ _ _ w241 _ _ _ _ _] -> w57
          tunnel: [_ _ _ _ _ w232 _ _ _ _ _] -> w56
          tunnel: [_ _ _ _ _ w233 _ _ _ _ _] -> w55
          tunnel: [_ _ _ _ _ w238 _ _ _ _ _] -> w54
          tunnel: [_ _ w133 _ _ _ _ _ _ _ _] -> w53
          tunnel: [_ _ w131 _ _ _ _ _ _ _ _] -> w52
          tunnel: [_ _ _ _ _ w230 _ _ _ _ _] -> w51
          tunnel: [_ _ w130 _ _ _ _ _ _ _ _] -> w50
          tunnel: [_ _ _ _ _ w229 _ _ _ _ _] -> w49
          frame #0 {
            w98 = FALSE ("Visible")
            w105 = TRUE ("Test Running 2")
            # "Init Controls"
            n22 = property class="App"() -> ("App.UserName"=w107:string)  [unwired: 2 in, 2 out]
            n23 = property on="Position" class="Str"("Visible"=FALSE) -> ()  [unwired: 2 in, 2 out]
            n24 = Unbundle By Name(w90) -> ("Log"=w104:refnum<class "Event Notification.lvclass">)
            n25 = local write "Operator"(w107) -> ()
            n26 = Unbundle By Name(w90) -> ("SW Rev.Version"=→"Rev":string)
            n27 = Unbundle By Name(w90) -> ("Cfg.Dirs.Logs"=w93:path)
            n28 = call <vilib>:"Event Notification.Status Message.vi"("Log"=TRUE, "Message"="Application Launched", "Event Notification in"=w104) -> ()  [unwired: 9 in]
            n29 = call "TestExec.Event Counter Log.vi"("Root Name"="Test Cycle Count", "Log Folder"=w93, "Read(T)/Inc and Save(F)"=TRUE ("Reset")) -> ("Event Cnt Out"=w94:i32)  [unwired: 8 in]
            n30 = local write "Total Test Cycles"(w94) -> ()
            n31 = invoke on="Pareto" class="Arr (strict)" method="Reinit To Default"() -> ()  [unwired: 3 in, 3 out]
            n32 = property on="Prompt2_OK" class="Bool"("Visible"=TRUE) -> ()  [unwired: 2 in, 2 out]
            n33 = property on="OperInput Data" class="Str"("Visible"=TRUE ("Key Focus")) -> ()  [unwired: 2 in, 2 out]
            n34 = property on="Prompt YES" class="Bool"("Visible"=w98) -> ()  [unwired: 2 in, 2 out]
            n35 = property on="Prompt NO" class="Bool"("Visible"=w98) -> ()  [unwired: 2 in, 2 out]
            n36 = property on="Test Running 2" class="Bool (strict)"("Blinking"=w105) -> ()  [unwired: 2 in, 2 out]
            "Status" <- "" ("Status")
            "Health OK" <- TRUE ("Health OK")
            "Test Running 2" <- w105
            "StaCnct" <- FALSE ("Sta")
            "Position" <- "" ("Pos")
            "Route Check" <- FALSE ("Route Check")
          }
          frame #1 {
            w114 = "Config" ("menu tag")
            # "This indicator is hidden unless in Sim mode."
            n37 = Unbundle By Name(w116) -> ("Cfg.Simulate"=w118:bool, "Menu Ref"=w113:refnum<k9>)
            n38 = Unbundle By Name(w116) -> ("Cfg.Is Child?"=w117:bool)
            n39 = case shown="True" w117 {
              tunnel: w113 -> [_ w125]
              frame False {
              }
              frame True {
                w127 = "Exit"
                n40 = Get Menu Item Info(7:w127, 11:w125) -> (0:w126:errorcluster, 2:w128:string, 3:w129:refnum<k9>)  [unwired: 1 in, 4 out]
                n41 = Set Menu Item Info(7:w127, 8:w126, 9:FALSE ("enabled"), 10:w128, 11:w129) -> (0:w123:errorcluster)  [unwired: 2 in, 1 out]
                n42 = call <vilib>:"Clear Errors.vi"("error in (no error)"=w123) -> ()  [unwired: 5 in, 2 out]
              }
            }
            n43 = property on="Simulate Indication" class="Str"("Visible"=w118) -> ()  [unwired: 2 in, 2 out]
            n44 = call <vilib>:"Menu.Simulate, Set Menu State.vi"("Sim Enable"=w118, "Menu Ref"=w113) -> ()  [unwired: 8 in, 2 out]
            n45 = property on="Test Status Tab" class="TabCtl (strict)"() -> ("Pages"=w110:refnum<vi>[])  [unwired: 2 in, 2 out]
            n46 = Set Menu Item Info(7:w114, 9:FALSE ("enabled"), 10:w114, 11:w113) -> ()  [unwired: 3 in, 2 out]
            n47 = for {
              tunnel: w110 -> [w122] mode=indexing
              tunnel: [w121] -> w111 mode=indexing
              tunnel: [w120] -> w112 mode=indexing
              n48 = property class="Page"(reference=w122) -> (reference out=w120:refnum<vi>, "PageLabel"=w121:string)  [unwired: 1 in, 1 out]
            }
            n49 = property on="Test Status Tab Sel" class="Ring (strict)"("Strings []"=w111) -> ()  [unwired: 2 in, 2 out]
            n50 = Close Reference(reference=w112) -> ()  [unwired: 1 in, 1 out]
            "Simulate Indication" <- "Simulate" ("Simulate Indication")
          }
          frame #2 {
            w130 = refnum<class "File.Sync.lvclass"> refnum  # Sync
            w131 = FALSE  # StaNotify
            w132 = 0.0  # SeqTimer
            w133 = cluster{"Seq":i32, "Name":string} {"Seq"=0, "Name"=""}  # Funct
            w134 = refnum<class "SeqMgr.lvclass"> refnum  # SeqMgr
            w135 = T22 {"Station Data"=[], "SeqRsltDirs"=[]}  # Data Dirs
            w136 = 0.0  # TimeOut(s)
            w137 = T65 {"Warnings"=0, "Errors"=0, "LastVerCk"=0.0, "VerCkInterval"=3600.0, "SW Check En"=FALSE, "Init"=FALSE, "LastVerListCk"=0.0}  # Health
            w138 = T63 {"State"=enum."Failing", "Code"=0, "Description"=""}  # ResultState
            w139 = string[][] []  # Seq
            w140 = T35 {"Oper"={"OK"=FALSE, "Desc"=""}, "SN"={"OK"=FALSE, "Desc"=""}, "NoSN"=FALSE, "DefaultSN"="", "SNErr"=FALSE, "SeqEn"=enum."Enabled"}  # PreTestCk
            w141 = T66[] []  # Sequences
            w142 = ""  # StaApp
            w144 = refnum<class "Mode Manager.lvclass"> refnum  # ModeMgr
            w143 = T67 {"ModeCfg"=path "C:/Users/ekaet/Dropbox/Valve/Source/MTE/MTE Testers/Applications/Test Executive/SubVIs/Mode Manager/Mode Manager.lvclass", "DataTemp"=path "", "SW Limits"=path "", "SW Sequences"=path "", "Rel_SW"=path "", "CurSeqDir"=path "", "RouteCfg"=path "", "WorkingCfg"=path "", "Devcon"=path "", "ScriptLibDirs"=[], "Archive"=path "", "LocalData"=path ""}  # CfgFilePaths
            w145 = TRUE  # Lnch
            # "Build Local Data Cluster"
          }
          frame #3 {
            w168 = T68 {"Child Modules"=[]}  # App
            # "TODO\nFwd Simulate to child"
            # "Launch Station Module"
            n51 = call "TestExec.Config, Get Station SW Module Info.vi"("Error if File Doesn't Exist"=TRUE) -> ("error out"=w156:errorcluster, "Station IP Port"=w152:i32, "Station Name"=w149:string)  [unwired: 7 in, 1 out]
            n52 = Unbundle By Name(w161) -> ("Cfg.Dirs"=w165:T27, "Cfg.Simulate"=w164:bool)
            n53 = Unbundle By Name(w161) -> ("SW Rev"=w166:T32)
            n54 = To Unsigned Word Integer(number=w152) -> (unsigned 16bit integer=w155:u16)
            n55 = Concatenate Strings("Sta_" ("string"), w149) -> (w146:string)
            "StaModule" <- w146
            n56 = Bundle By Name(cluster=T34 {"IP"="127.0.0.1", "Port"=8500, "Listener"=FALSE, "Enable"=FALSE} ("Config"), "Port"=w155, "Listener"=FALSE, "Enable"=TRUE) -> (w150:T34)
            n57 = case shown="No Error" w156 {
              selector: w156 -> [_ w206]
              tunnel: w166 -> [w182 _]
              tunnel: w165 -> [w180 _]
              tunnel: w164 -> [w179 _]
              tunnel: w163 -> [w178 _]
              tunnel: [w177 _] -> w162
              tunnel: [w176 w206] -> w158
              tunnel: w150 -> [w174 _]
              tunnel: w146 -> [w173 _]
              frame No Error {
                n58 = for {
                  N: 2 -> [_]
                  tunnel: w182 -> [w191]
                  tunnel: [w186] -> w177 mode=indexing
                  tunnel: w178 -> [w189]
                  tunnel: w180 -> [w188]
                  tunnel: w179 -> [w187]
                  tunnel: [w185] -> w175 mode=indexing
                  tunnel: w174 -> [w184]
                  tunnel: w173 -> [w183]
                  i -> [w190]
                  n59 = case shown="0, Default" w190 {
                    tunnel: w191 -> [_ _]
                    tunnel: w189 -> [w199 _]
                    tunnel: w188 -> [_ _]
                    tunnel: w187 -> [_ _]
                    tunnel: [w201 w204] -> w186
                    tunnel: [w200 _] -> w185
                    tunnel: w184 -> [w197 _]
                    tunnel: w183 -> [w192 _]
                    frame 0, Default {
                      n60 = control-ref of="StaCnct"() -> (w196:refnum<vi>)
                      n61 = call <vilib>:"Q.Obtain Queue.vi"("Q Name"=w192) -> ("Q Out"=w198:refnum<queue>)  [unwired: 8 in, 2 out]
                      n62 = call <vilib>:"TCP-IP Q_Bridge.Create.vi"("Auto Exit"=TRUE, "Notification"=TRUE, "Config"=w197, "StatusCtrlRef"=w196, "Q_DataOut"=w198, "Q_DataIn"=w199, "Control Q Name"="TCP-IP_TE") -> ("Error Out"=w200:errorcluster)  [unwired: 3 in, 1 out]
                      n63 = Bundle By Name(cluster=cluster{"VI Ref":refnum<vi>, "Name":string} {"VI Ref"=refnum, "Name"=""} ("output cluster"), "Name"=w192) -> (w201:cluster{"VI Ref":refnum<vi>, "Name":string})
                    }
                    frame 1 {
                      n64 = Bundle By Name(cluster=cluster{"VI Ref":refnum<vi>, "Name":string} {"VI Ref"=refnum, "Name"=""} ("output cluster"), "Name"="Wiggler" ("Q Name")) -> (w204:cluster{"VI Ref":refnum<vi>, "Name":string})
                    }
                  }
                }
                n65 = Merge Errors(w175) -> (w176:errorcluster)
              }
              frame Error {
              }
            }
            n66 = Bundle By Name(cluster=w168, "Child Modules"=w162) -> (w167:T68)
            n67 = case shown="Error" w158 {
              selector: w158 -> [w169 _]
              tunnel: -5000 ("Code(0 = no change)") -> [_ w172]
              tunnel: "Test Exec error launching TCP-IP for Station" ("Description") -> [_ w171]
              tunnel: [w169 w170] -> w157
              frame No Error {
              }
              frame Error {
                n68 = call "Error.Set-Change Error Info.vi"("Description"=w171, "Cust Code(0 = no change)"=w172) -> ("error out"=w170:errorcluster)  [unwired: 9 in]
              }
            }
          }
          frame #4 {
            # "Add persisten controls here"
            # "Restore saved control states"
            n69 = while {
              shift-right: [w215] -> w209
              shift-left: refnum<vi>[] [] -> [w216]
              i -> [w217]
              stop <- w214 stop-if-true
              n70 = case shown="0" w217 {
                tunnel: w216 -> [w225 w228]
                tunnel: [w226 w228] -> w215
                tunnel: [_ TRUE] -> w214
                frame 0 {
                  w219 = refnum<vi> refnum  # Control
                  n71 = control-ref of="Log Level"() -> (w221:refnum<vi>)
                  n72 = control-ref of="SyncType"() -> (w220:refnum<vi>)
                  n73 = control-ref of="Period"() -> (w223:refnum<vi>)
